vi "AD5781StepLogic.vi"(4 "actTrack":i32, 6 "actStep":i32) -> (2 "timedOut":bool)   [LabVIEW 2014]
uses:
  Sequencer/trackGlobVar.vi
  <vilib>/rvi/Emulation/niFpgaGetClockAttributes.vi
  <vilib>/rvi/Emulation/niFpgaSctlEmulationGetInTimedLoop.vi
  <vilib>/rvi/Emulation/niFpgaEmulationReportErrorSimple.vi
  <vilib>/rvi/Emulation/niFpgaCriticalErrorInLSC.vi
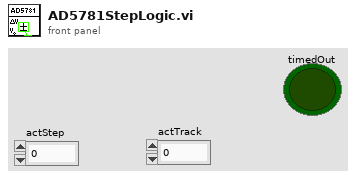
[diagram p1: front panel]
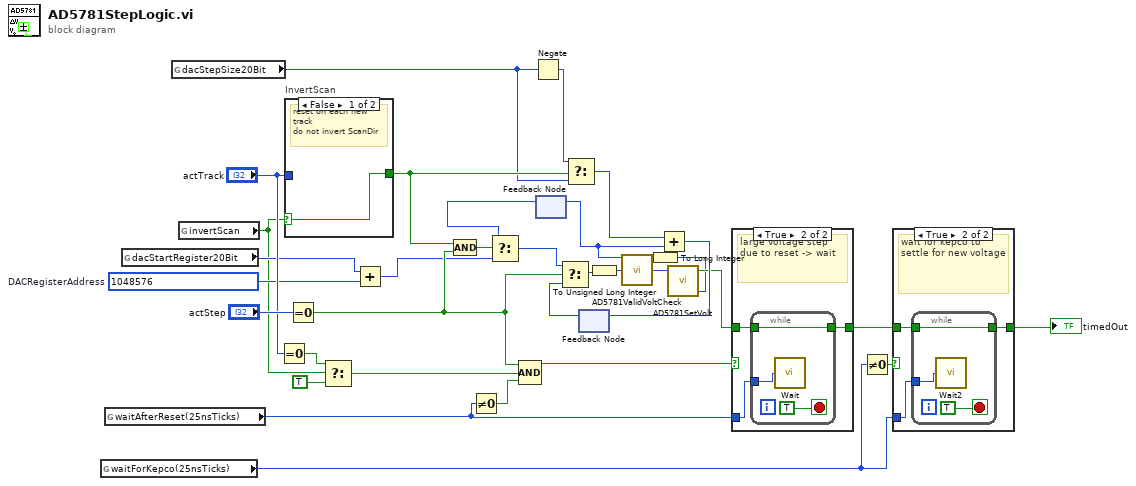
[diagram p0: block diagram]
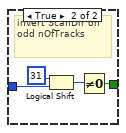
[diagram p3: hidden frame]
diagram:
  w6 = 1048576  # DACRegisterAddress
  n1 = global read "trackGlobVar.vi" "waitForKepco(25nsTicks)"() -> (w1:u16)
  n2 = global read "trackGlobVar.vi" "waitAfterReset(25nsTicks)"() -> (w2:u16)
  n3 = global read "trackGlobVar.vi" "dacStartRegister20Bit"() -> (w4:i32)
  n4 = global read "trackGlobVar.vi" "dacStepSize20Bit"() -> (w5:i32)
  n5 = global read "trackGlobVar.vi" "invertScan"() -> (w3:bool)
  n6 = Equal To 0?(x="actTrack") -> (x = 0?=w18:bool)
  n7 = case "InvertScan" shown="False" w3 {
    selector: w3 -> [w33 _]
    tunnel: [w33 w34] -> w19
    tunnel: "actTrack" -> [_ w37]
    frame False {
      # "reset on each new track\ndo not invert ScanDir"
    }
    frame True {
      # "invert ScanDir on odd nOfTracks"
      n8 = Logical Shift(y=i16 31, x=w37) -> (x << y=w35:i32)
      n9 = Not Equal To 0?(x=w35) -> (x != 0?=w34:bool)
    }
  }
  n10 = Equal To 0?(x="actStep") -> (x = 0?=w21:bool)
  n11 = Select(t=w18, s=w3, f=TRUE) -> (s? t:f=w16:bool)
  n12 = Add(x=w4, y=w6) -> (x+y=w7:i32)
  n13 = Compound Arithmetic op=AND(w19, w21) -> (w26:bool)
  n14 = Not Equal To 0?(x=w2) -> (x != 0?=w15:bool)
  n15 = Compound Arithmetic op=AND(w21, w16, w15) -> (w24:bool)
  n16 = Negate(x=w5) -> (-x=w32:i32)
  n17 = feedback #1() -> (w25:i32)  [unwired: 1 in]
  n18 = Select(t=w25, s=w26, f=w7) -> (s? t:f=w27:i32)
  n19 = Select(t=w32, s=w19, f=w5) -> (s? t:f=w31:i32)
  n20 = feedback #2() -> (w29:i32)  [unwired: 1 in]
  n21 = Select(t=w27, s=w21, f=w29) -> (s? t:f=w23:i32)
  n22 = To Unsigned Long Integer(number=w23) -> (unsigned 32bit integer=w9:u32)
  n23 = call "AD5781ValidVoltCheck.vi"("U32"=w9) -> ("coerced(x)"=w8:u32)  [unwired: 4 in]
  n24 = call "AD5781SetVolt.vi"("SetVolt"=w8) -> ("Readback"=w11:u32, "timedOut"=w28:bool)  [unwired: 2 in, 1 out]
  n25 = To Long Integer(number=w11) -> (32bit integer=w10:i32)
  n26 = feedback-in #1(w10) -> ()
  n27 = Add(x=w31, y=w10) -> (x+y=w30:i32)
  n28 = feedback-in #2(w30) -> ()
  n29 = case shown="True" w24 {
    tunnel: w28 -> [w38 w41]
    tunnel: [w38 w40] -> w14
    tunnel: w2 -> [_ w39]
    frame False {
    }
    frame True {
      # "large voltage step due to reset -> wait"
      n30 = while {
        tunnel: w41 -> [w43]
        tunnel: [w43] -> w40
        tunnel: w39 -> [w42]
        stop <- TRUE stop-if-true
        n31 = call "Wait"("Count(Ticks)"=w42) -> ()  [unwired: 1 out]
      }
    }
  }
  n32 = Not Equal To 0?(x=w1) -> (x != 0?=w13:bool)
  n33 = case shown="True" w13 {
    tunnel: w14 -> [w45 w48]
    tunnel: [w45 w47] -> w12
    tunnel: w1 -> [_ w46]
    frame False {
    }
    frame True {
      # "wait for kepco to settle for new voltage"
      n34 = while {
        tunnel: w48 -> [w50]
        tunnel: [w50] -> w47
        tunnel: w46 -> [w49]
        stop <- TRUE stop-if-true
        n35 = call "Wait2"("Count(Ticks)"=w49) -> ()  [unwired: 1 out]
      }
    }
  }
  "timedOut" <- w12
